vi "Camera Global.vi"() -> ()   [LabVIEW 2016]
panel:
  out "cameraStatus":bool
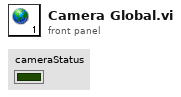
[diagram p1: front panel]
diagram:
